vi "Load_VI.vi"   [LabVIEW 2025]
uses:
  <vilib>/ActorFramework/Actor/Actor.lvclass
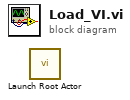
[diagram p0: block diagram]
diagram:
  n1 = call <vilib>:"Launch Root Actor.vi"() -> ()  [unwired: 10 in, 2 out]
